vi "Add Hierarchy.vi"(8 "error in (no error)":errorcluster, 10 "Hierarchy":T1[](array[typedef]), 11 "Security in":refnum<class "Security.lvclass">) -> (0 "error out":errorcluster, 3 "Security out":refnum<class "Security.lvclass">)   [LabVIEW 2020, in "HTTP Server.lvlib" / "Security.lvclass"]
uses:
  Security.lvclass
  Role Inheritance.ctl
  Security.lvclass/Security.ctl
  <vilib>/Utility/miscctls.llb/LVMapReplaceAction.ctl
  HTTP Server.lvlib
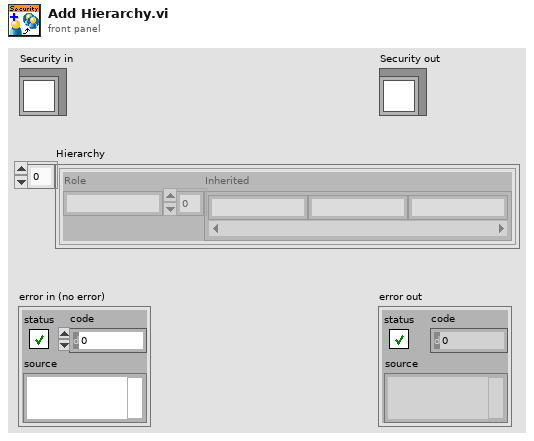
[diagram p1: front panel]
types:
  T1 = typedef "HTTP Server.lvlib/Role Inheritance.ctl" = cluster{"Role":string, "Inherited":string[]}
  T2 = typedef "LVMapReplaceAction.ctl" = enum32{"Modify Entry only if found", "Add or Modify Entry", "Delete Entry"}
  T3 = typedef "HTTP Server.lvlib/Security.lvclass/Ref Data.ctl" = cluster{"Hierarchy":T4}
  T4 = typedef "HTTP Server.lvlib/Security.lvclass/Hierarchy.ctl" = map{string, set{string}}
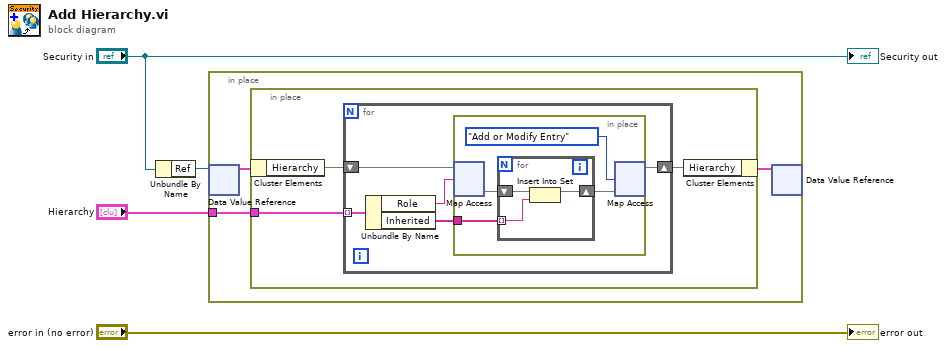
[diagram p0: block diagram]
diagram:
  n1 = Unbundle By Name("Security in") -> ("Ref"=w3:refnum<data-value>)
  n2 = in-place {
    in-place-border: "Hierarchy" -> [w5]
    n3 = in-place-dvr #1(w3) -> (w7:T3)  [unwired: 1 out]
    n4 = in-place {
      in-place-border: w5 -> [w10]
      n5 = in-place-cluster #2(w7) -> ("Hierarchy"=w9:T4)
      n6 = for {
        tunnel: w10 -> [w15] mode=indexing
        shift-right: [w11] -> w8
        shift-left: w9 -> [w14]
        n7 = Unbundle By Name(w15) -> ("Role"=w13:string, "Inherited"=w12:string[])
        n8 = in-place {
          in-place-border: w12 -> [w18]
          n9 = in-place-map #3(w14, w13) -> (w19:set{string})  [unwired: 1 in, 1 out]
          n10 = for {
            shift-right: [w20] -> w17
            shift-left: w19 -> [w22]
            tunnel: w18 -> [w21] mode=indexing
            n11 = Insert Into Set(10:w21, 11:w22) -> (3:w20:set{string})  [unwired: 1 out]
          }
          n12 = in-place-map #3(w17, LVMapReplaceAction."Add or Modify Entry" ("action")) -> (w11:T4)  [unwired: 2 out]
        }
      }
      n13 = in-place-cluster #2("Hierarchy"=w8) -> (w6:T3)
    }
    n14 = in-place-dvr #1(w6) -> ()  [unwired: 2 out]
  }
  "error out" <- "error in (no error)"
  "Security out" <- "Security in"
